vi "Init Condition.vi"(5 "Sequencing":refnum<class "MessageQ.lvclass">, 6 "Variables":refnum<class "Variables.lvclass">, 7 "VolatusAPI":refnum<class "VolatusAPI.lvclass">, 8 "error in (no error)":refnum<class "MultiErrors.lvclass">, 10 "Condition Config":refnum<class "Condition Config.lvclass">, 11 "Condition in":refnum<class "Condition.lvclass">) -> (0 "error out":refnum<class "MultiErrors.lvclass">, 3 "Condition out":refnum<class "Condition.lvclass">)   [LabVIEW 2020, in "VolatusSeq.lvlib" / "Condition.lvclass"]
uses:
  Condition.lvclass
  VolatusErrorUtilities/MultiErrors/MultiErrors.lvclass
  Volatus/VolatusAPI/VolatusAPI.lvclass
  VolatusSeqConfig/Condition Config/Condition Config.lvclass
  Volatus/MessageQ/MessageQ.lvclass
  Condition.lvclass/Condition.ctl
  Variables/Variables.lvclass
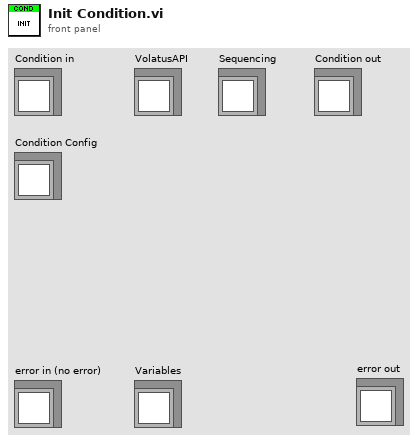
[diagram p1: front panel]
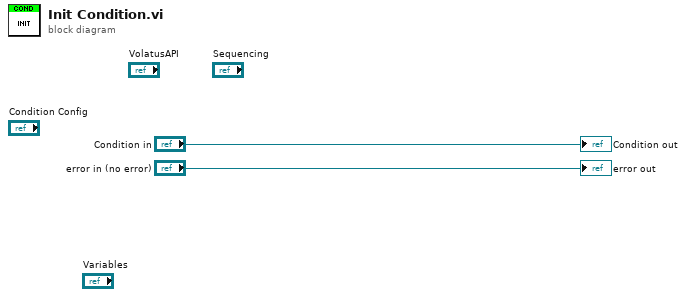
[diagram p0: block diagram]
diagram:
  "error out" <- "error in (no error)"
  "Condition out" <- "Condition in"
